vi "Get Drive Information.vi"() -> (0 "Ticks/Revolution":dbl, 3 "Wheel Diameter":dbl)   [LabVIEW 2019]
doc: "Wheel diameter and encoder information for different drive bases. Useful for pathplanning."
panel:
  in  "Robot":enum16{"Vantage", "Mule"}(ring)
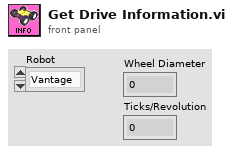
[diagram p1: front panel]
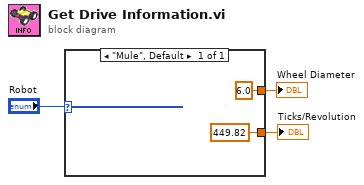
[diagram p0: block diagram]
diagram:
  n1 = case shown="\"Mule\", Default" "Robot" {
    tunnel: [6.0 ("x")] -> w3
    tunnel: [449.82 ("y")] -> w2
    frame "Mule", Default {
    }
  }
  "Wheel Diameter" <- w3
  "Ticks/Revolution" <- w2
